vi "MKS VI Probe.vi"() -> ()   [LabVIEW 2015]
doc: "Example VI that demonstrates all library features."
uses:
  PL MKS VI Probe.lvclass
panel:
  in  "baud rate":u32(ring)=19200 items=["300"=300, "600"=600, "1200"=1200, "2400"=2400, "4800"=4800, "9600"=9600, "19200"=19200, "38400"=38400, "76800"=76800, "115200"=115200]
  in  "read software revision":bool
  out "Preact, var":dbl
  out "Pact, W":dbl
  out "Prev, W":dbl
  out "Pfwd, W":dbl
  out "|Z|, Ohm":dbl
  out "Irms, A":dbl
  out "Urms, V":dbl
  out "phase, °":dbl
  in  "save parameters to EEPROM":bool
  out "frequency scan in progress":bool
  in  "Tab Control":enum32{"Frequency scan", "FFT", "Waveforms"}(tab)
  in  "frequency scan parameters":enum32{"range", "array"}(tab)
  in  "frequency range":T1={"start, Hz"=1000000, "stop, Hz"=10000000, "step, Hz"=1000000} {"step, Hz" format="%.0p"; "stop, Hz" format="%.0p"; "start, Hz" format="%.0p"}
  in  "frequency array":u32[](array[numeric]) format="%.0p"
  in  "frequency scan":bool
  out "frequency scan graph":cluster{u32[], dbl[]}[](graph)
  out "frequency scan timeout, ms":u32
  in  "read FFT":bool
  out "FFT graph":T2(graph)
  in  "read waveforms":bool
  out "waveform graph":T3(graph)
  in  "buffers":u16(ring) items=["all on", "oscilloscope on", "spectrum on", "all off"]
  in  "acquisition time, ms":u16(ring) items=["4.08", "6.08", "12.20", "20.96", "42.61", "85.20", "170.40", "348.60", "687.20"]
  in  "averaging":u16(ring) items=["1", "2", "4", "8", "16", "32", "64", "128"]
  in  "end address":u32
  in  "start address":u32
  in  "frequency, Hz":u32=1000000 format="%.0p"
  in  "read firmware checksum":bool
  out "VI Probe":refnum<class "PL MKS VI Probe.lvclass">
  in  "port":refnum<visa-resource-name>
  out "error":errorcluster
  in  "stop":bool
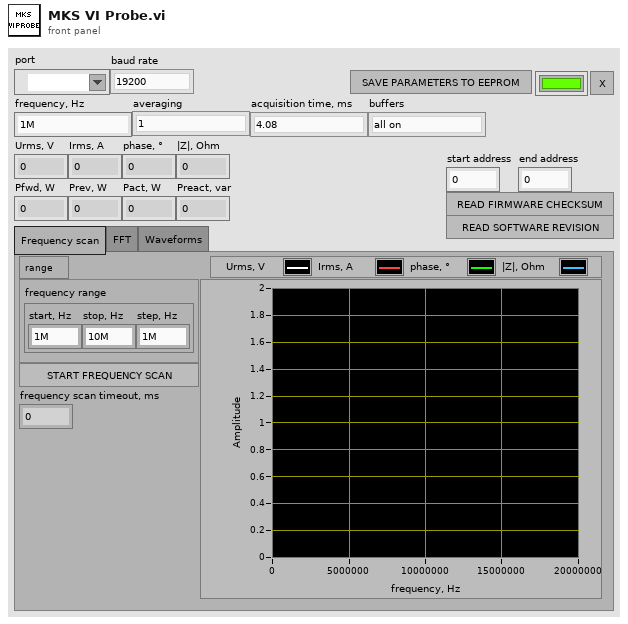
[diagram p1: front panel]
types:
  T1 = cluster{"start, Hz":u32, "stop, Hz":u32, "step, Hz":u32}
  T2 = cluster{"f, Hz":dbl, "df, Hz":dbl, "magnitude, dB":dbl[][]}
  T3 = cluster{"t0, s":dbl, "dt, s":dbl, "U, V":dbl[][]}
  T4 = cluster{"frequency, Hz":u32, "time, s":dbl, "status":cluster{"rf on":bool, "time overflow":bool, "avarage data valid":bool, "below scan threshold":bool, "computational overflow":bool}, "Urms, V":dbl, "Irms, A":dbl, "phase difference, °":dbl, "|Z|, Ohm":dbl}
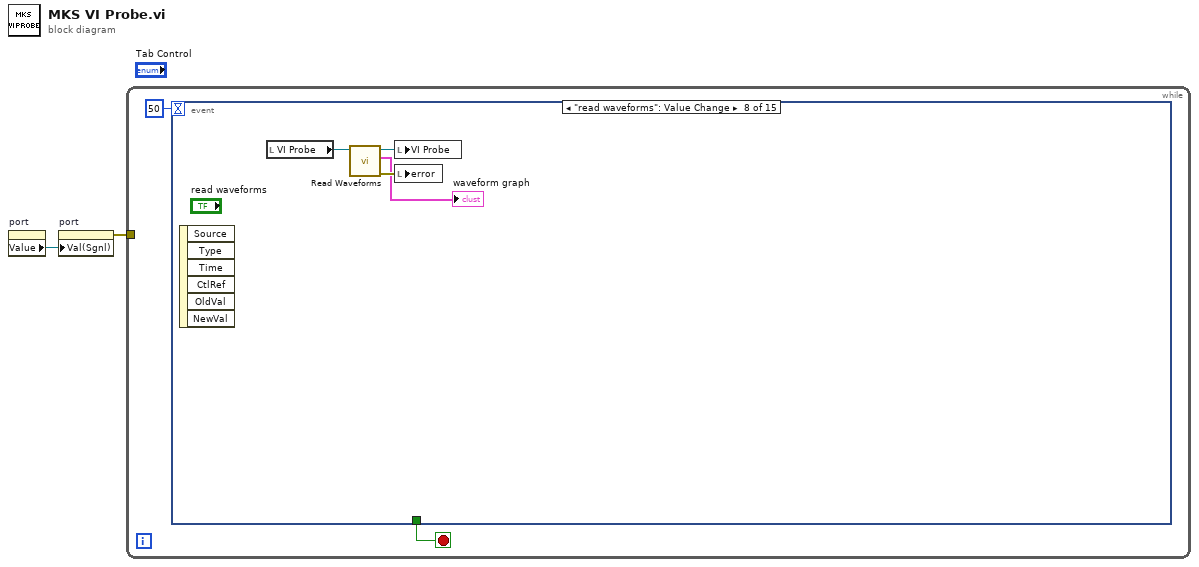
[diagram p0: block diagram]
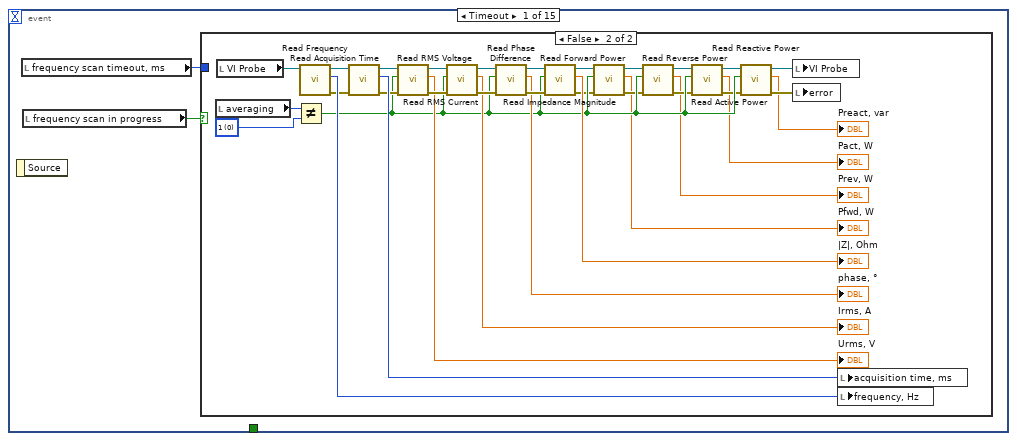
[diagram p2: hidden frame]
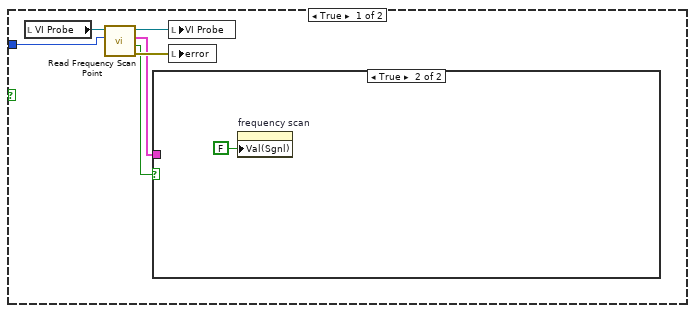
[diagram p3: hidden frame]
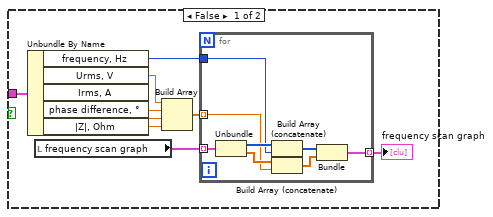
[diagram p4: hidden frame]
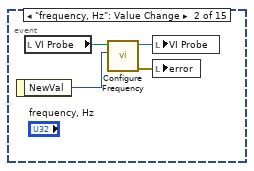
[diagram p5: hidden frame]
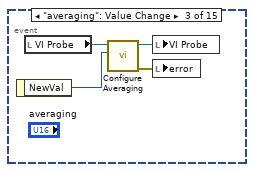
[diagram p6: hidden frame]
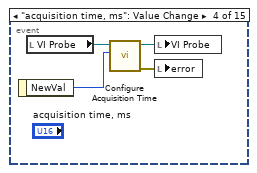
[diagram p7: hidden frame]
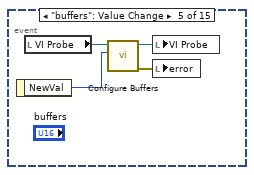
[diagram p8: hidden frame]
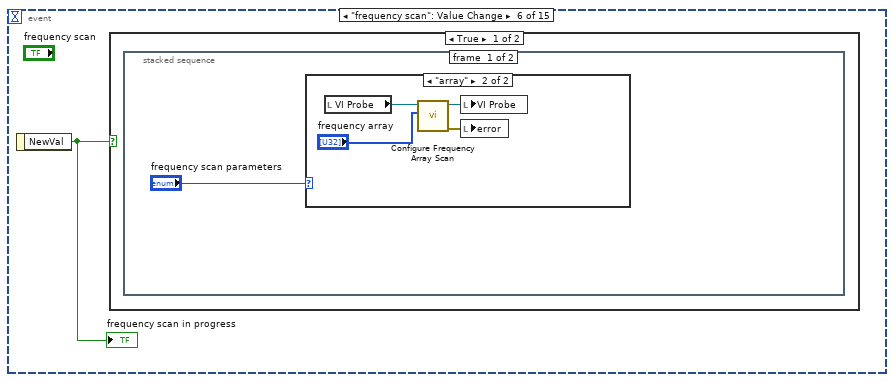
[diagram p9: hidden frame]
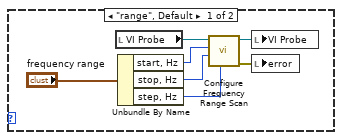
[diagram p10: hidden frame]
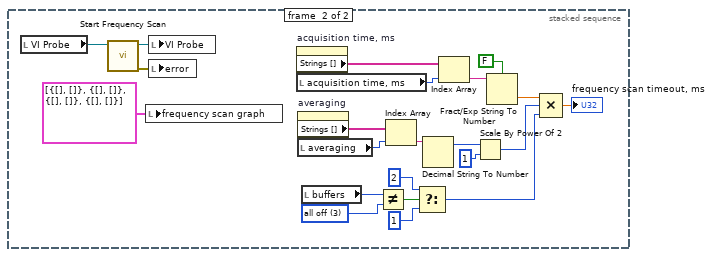
[diagram p11: hidden frame]
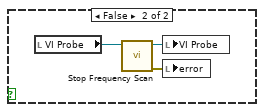
[diagram p12: hidden frame]
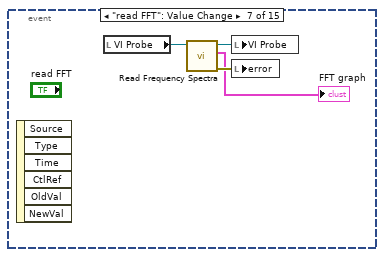
[diagram p13: hidden frame]
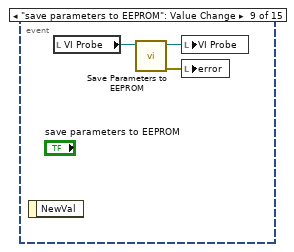
[diagram p14: hidden frame]
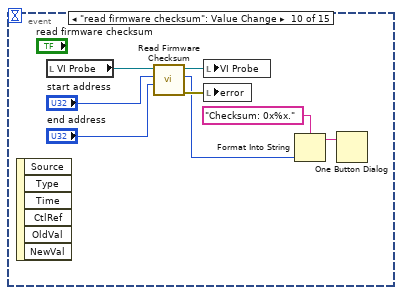
[diagram p15: hidden frame]
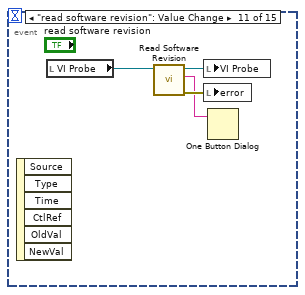
[diagram p16: hidden frame]
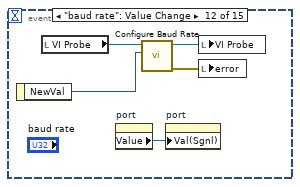
[diagram p17: hidden frame]
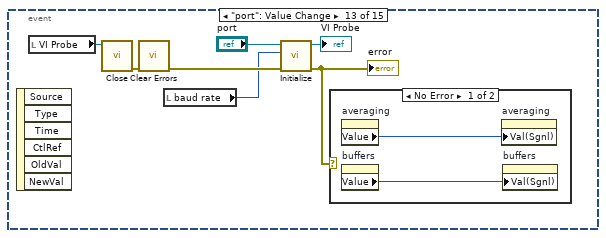
[diagram p18: hidden frame]
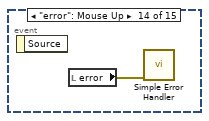
[diagram p20: hidden frame]
diagram:
  n1 = property on="port" class="VISAName"() -> ("Value"=w1:refnum<visa-resource-name>)  [unwired: 2 in, 2 out]
  n2 = property on="port" class="VISAName"("Val(Sgnl)"=w1) -> (error out=w2:errorcluster)  [unwired: 2 in, 1 out]
  n3 = while {
    tunnel: w2 -> [_]
    stop <- w3 stop-if-true
    n4 = event shown="[7] \"read waveforms\": Value Change" {
      selector: _ -> [_ _ _ _ _ _ _ _ _ _ _ _ _ _ _]
      dyn-events: _ -> [_ _ _ _ _ _ _ _ _ _ _ _ _ _ _]
      timeout: 50 -> [_ _ _ _ _ _ _ _ _ _ _ _ _ _ _]
      tunnel: [_ _ _ _ _ _ _ _ _ _ _ _ _ _ TRUE ("stop")] -> w3
      event Timeout {
        n5 = event-data() -> ()  [unwired: 1 in, 1 out]
        n6 = local read "frequency scan timeout, ms"() -> (w5:u32)
        n7 = local read "frequency scan in progress"() -> (w6:bool)
        n8 = case shown="False" w6 {
          tunnel: w5 -> [w9 _]
          frame True {
            n9 = local read "VI Probe"() -> (w12:refnum<class "PL MKS VI Probe.lvclass">)
            n10 = call "Read Frequency Scan Point.vi"("additional timeout, ms (0)"=w9, "VI Probe in"=w12) -> ("error out"=w10:errorcluster, "end of scan"=w7:bool, "scan point"=w8:T4, "VI Probe out"=w11:refnum<class "PL MKS VI Probe.lvclass">)  [unwired: 6 in]
            n11 = case shown="True" w7 {
              tunnel: w8 -> [w21 _]
              frame False {
                n12 = Unbundle By Name(w21) -> ("frequency, Hz"=w14:u32, "Urms, V"=w19:dbl, "Irms, A"=w18:dbl, "phase difference, °"=w17:dbl, "|Z|, Ohm"=w16:dbl)
                n13 = local read "frequency scan graph"() -> (w20:cluster{u32[], dbl[]}[])
                n14 = Build Array(w19, w18, w17, w16) -> (w15:dbl[])
                n15 = for {
                  tunnel: w20 -> [w29] mode=indexing
                  tunnel: w15 -> [w25] mode=indexing
                  tunnel: w14 -> [w26]
                  tunnel: [w22] -> w13 mode=indexing
                  n16 = Unbundle(w29) -> (w28:u32[], w27:dbl[])
                  n17 = Build Array (concatenate)(w28, w26) -> (w24:u32[])
                  n18 = Build Array (concatenate)(w27, w25) -> (w23:dbl[])
                  n19 = Bundle(w24, w23) -> (w22:cluster{u32[], dbl[]})  [unwired: 1 in]
                }
                "frequency scan graph" <- w13
              }
              frame True {
                n20 = property on="frequency scan" class="Bool (strict)"("Val(Sgnl)"=FALSE ("Value (Signaling)")) -> ()  [unwired: 2 in, 2 out]
              }
            }
            n21 = local write "VI Probe"(w11) -> ()
            n22 = local write "error"(w10) -> ()
          }
          frame False {
            w59 = u16 0 items=["1", "2", "4", "8", "16", "32", "64", "128"] ("averaging")
            n23 = local read "averaging"() -> (w58:u16)
            n24 = local read "VI Probe"() -> (w64:refnum<class "PL MKS VI Probe.lvclass">)
            n25 = Not Equal?(x=w58, y=w59) -> (x != y?=w45:bool)
            n26 = call "Read Frequency.vi"("VI Probe in"=w64) -> ("error out"=w61:errorcluster, "frequency, Hz"=w63:u32, "VI Probe out"=w62:refnum<class "PL MKS VI Probe.lvclass">)  [unwired: 8 in]
            n27 = call "Read Acquisition Time.vi"("error in (no error)"=w61, "VI Probe in"=w62) -> ("error out"=w50:errorcluster, "acquisition time, ms"=w60:u16, "VI Probe out"=w57:refnum<class "PL MKS VI Probe.lvclass">)  [unwired: 7 in]
            n28 = call "Read RMS Voltage.vi"("error in (no error)"=w50, "average (false)"=w45, "VI Probe in"=w57) -> ("error out"=w51:errorcluster, "Urms, V"=→"Urms, V":dbl, "VI Probe out"=w56:refnum<class "PL MKS VI Probe.lvclass">)  [unwired: 6 in]
            n29 = call "Read RMS Current.vi"("error in (no error)"=w51, "average (false)"=w45, "VI Probe in"=w56) -> ("error out"=w52:errorcluster, "Irms, A"=→"Irms, A":dbl, "VI Probe out"=w55:refnum<class "PL MKS VI Probe.lvclass">)  [unwired: 6 in]
            n30 = call "Read Phase Difference.vi"("error in (no error)"=w52, "average (false)"=w45, "VI Probe in"=w55) -> ("error out"=w53:errorcluster, "phase difference, °"=→"phase, °":dbl, "VI Probe out"=w54:refnum<class "PL MKS VI Probe.lvclass">)  [unwired: 6 in]
            n31 = call "Read Impedance Magnitude.vi"("error in (no error)"=w53, "average (false)"=w45, "VI Probe in"=w54) -> ("error out"=w35:errorcluster, "|Z|, Ohm"=→"|Z|, Ohm":dbl, "VI Probe out"=w44:refnum<class "PL MKS VI Probe.lvclass">)  [unwired: 6 in]
            n32 = call "Read Forward Power.vi"("error in (no error)"=w35, "average (false)"=w45, "VI Probe in"=w44) -> ("error out"=w36:errorcluster, "Pfwd, W"=→"Pfwd, W":dbl, "VI Probe out"=w43:refnum<class "PL MKS VI Probe.lvclass">)  [unwired: 6 in]
            n33 = call "Read Reverse Power.vi"("error in (no error)"=w36, "average (false)"=w45, "VI Probe in"=w43) -> ("error out"=w37:errorcluster, "Prev, W"=→"Prev, W":dbl, "VI Probe out"=w42:refnum<class "PL MKS VI Probe.lvclass">)  [unwired: 6 in]
            n34 = call "Read Active Power.vi"("error in (no error)"=w37, "average (false)"=w45, "VI Probe in"=w42) -> ("error out"=w38:errorcluster, "Pact, W"=→"Pact, W":dbl, "VI Probe out"=w41:refnum<class "PL MKS VI Probe.lvclass">)  [unwired: 6 in]
            n35 = call "Read Reactive Power.vi"("error in (no error)"=w38, "average (false)"=w45, "VI Probe in"=w41) -> ("error out"=w39:errorcluster, "Preact, var"=→"Preact, var":dbl, "VI Probe out"=w40:refnum<class "PL MKS VI Probe.lvclass">)  [unwired: 6 in]
            n36 = local write "VI Probe"(w40) -> ()
            n37 = local write "error"(w39) -> ()
            n38 = local write "acquisition time, ms"(w60) -> ()
            n39 = local write "frequency, Hz"(w63) -> ()
          }
        }
      }
      event "frequency, Hz": Value Change {
        n40 = event-data() -> ("NewVal"=w65:u32)  [unwired: 1 in]
        n41 = local read "VI Probe"() -> (w68:refnum<class "PL MKS VI Probe.lvclass">)
        n42 = call "Configure Frequency.vi"("frequency, Hz"=w65, "VI Probe in"=w68) -> ("error out"=w66:errorcluster, "VI Probe out"=w67:refnum<class "PL MKS VI Probe.lvclass">)  [unwired: 8 in]
        n43 = local write "VI Probe"(w67) -> ()
        n44 = local write "error"(w66) -> ()
      }
      event "averaging": Value Change {
        n45 = event-data() -> ("NewVal"=w69:u16)  [unwired: 1 in]
        n46 = local read "VI Probe"() -> (w72:refnum<class "PL MKS VI Probe.lvclass">)
        n47 = call "Configure Averaging.vi"("number of points"=w69, "VI Probe in"=w72) -> ("error out"=w70:errorcluster, "VI Probe out"=w71:refnum<class "PL MKS VI Probe.lvclass">)  [unwired: 8 in]
        n48 = local write "VI Probe"(w71) -> ()
        n49 = local write "error"(w70) -> ()
      }
      event "acquisition time, ms": Value Change {
        n50 = event-data() -> ("NewVal"=w73:u16)  [unwired: 1 in]
        n51 = local read "VI Probe"() -> (w76:refnum<class "PL MKS VI Probe.lvclass">)
        n52 = call "Configure Acquisition Time.vi"("acquisition time, ms"=w73, "VI Probe in"=w76) -> ("error out"=w74:errorcluster, "VI Probe out"=w75:refnum<class "PL MKS VI Probe.lvclass">)  [unwired: 8 in]
        n53 = local write "VI Probe"(w75) -> ()
        n54 = local write "error"(w74) -> ()
      }
      event "buffers": Value Change {
        n55 = event-data() -> ("NewVal"=w77:u16)  [unwired: 1 in]
        n56 = local read "VI Probe"() -> (w80:refnum<class "PL MKS VI Probe.lvclass">)
        n57 = call "Configure Buffers.vi"("mode"=w77, "VI Probe in"=w80) -> ("error out"=w78:errorcluster, "VI Probe out"=w79:refnum<class "PL MKS VI Probe.lvclass">)  [unwired: 8 in]
        n58 = local write "VI Probe"(w79) -> ()
        n59 = local write "error"(w78) -> ()
      }
      event "frequency scan": Value Change {
        n60 = event-data() -> ("NewVal"=w81:bool)  [unwired: 1 in]
        "frequency scan in progress" <- w81
        n61 = case shown="True" w81 {
          frame True {
            n62 = stacked-sequence {
              frame #0 {
                n63 = case shown="\"array\"" "frequency scan parameters" {
                  frame "range", Default {
                    n64 = local read "VI Probe"() -> (w88:refnum<class "PL MKS VI Probe.lvclass">)
                    n65 = Unbundle By Name("frequency range") -> ("start, Hz"=w87:u32, "stop, Hz"=w86:u32, "step, Hz"=w85:u32)
                    n66 = call "Configure Frequency Range Scan.vi"("step, Hz"=w85, "stop, Hz"=w86, "start, Hz"=w87, "VI Probe in"=w88) -> ("error out"=w84:errorcluster, "VI Probe out"=w83:refnum<class "PL MKS VI Probe.lvclass">)  [unwired: 6 in]
                    n67 = local write "VI Probe"(w83) -> ()
                    n68 = local write "error"(w84) -> ()
                  }
                  frame "array" {
                    n69 = local read "VI Probe"() -> (w93:refnum<class "PL MKS VI Probe.lvclass">)
                    n70 = call "Configure Frequency Array Scan.vi"("frequencies, Hz"="frequency array", "VI Probe in"=w93) -> ("error out"=w92:errorcluster, "VI Probe out"=w91:refnum<class "PL MKS VI Probe.lvclass">)  [unwired: 8 in]
                    n71 = local write "VI Probe"(w91) -> ()
                    n72 = local write "error"(w92) -> ()
                  }
                }
              }
              frame #1 {
                w95 = u16 3 items=["all on", "oscilloscope on", "spectrum on", "all off"] ("buffers")
                n73 = local read "VI Probe"() -> (w114:refnum<class "PL MKS VI Probe.lvclass">)
                n74 = call "Start Frequency Scan.vi"("VI Probe in"=w114) -> ("error out"=w112:errorcluster, "VI Probe out"=w113:refnum<class "PL MKS VI Probe.lvclass">)  [unwired: 9 in]
                n75 = local write "frequency scan graph"(cluster{u32[], dbl[]}[] [{[], []}, {[], []}, {[], []}, {[], []}] ("frequency scan graph")) -> ()
                n76 = local write "VI Probe"(w113) -> ()
                n77 = local write "error"(w112) -> ()
                n78 = property on="acquisition time, ms" class="Ring (strict)"() -> ("Strings []"=w104:string[])  [unwired: 2 in, 2 out]
                n79 = local read "acquisition time, ms"() -> (w105:u16)
                n80 = property on="averaging" class="Ring (strict)"() -> ("Strings []"=w99:string[])  [unwired: 2 in, 2 out]
                n81 = local read "averaging"() -> (w100:u16)
                n82 = local read "buffers"() -> (w94:u16)
                n83 = Not Equal?(x=w94, y=w95) -> (x != y?=w96:bool)
                n84 = Index Array(array=w99, index=w100) -> (element=w101:string)
                n85 = Select(t=u32 2 ("additional timeout, ms (0)"), s=w96, f=u32 1 ("additional timeout, ms (0)")) -> (s? t:f=w110:u32)
                n86 = Decimal String To Number(string=w101) -> (offset past number=w102:i32)  [unwired: 2 in, 1 out]
                n87 = Index Array(array=w104, index=w105) -> (element=w106:string)
                n88 = Scale By Power Of 2(n=w102, x=u32 1) -> (x*2^n=w109:u32)
                n89 = Fract/Exp String To Number(use system decimal point (T)=FALSE, string=w106) -> (number=w108:dbl)  [unwired: 2 in, 1 out]
                n90 = Compound Arithmetic op=MULTIPLY(w108, w109, w110) -> (→"frequency scan timeout, ms":dbl)
              }
            }
          }
          frame False {
            n91 = local read "VI Probe"() -> (w118:refnum<class "PL MKS VI Probe.lvclass">)
            n92 = call "Stop Frequency Scan.vi"("VI Probe in"=w118) -> ("error out"=w116:errorcluster, "VI Probe out"=w117:refnum<class "PL MKS VI Probe.lvclass">)  [unwired: 9 in]
            n93 = local write "VI Probe"(w117) -> ()
            n94 = local write "error"(w116) -> ()
          }
        }
      }
      event "read FFT": Value Change {
        n95 = event-data() -> ()  [unwired: 1 in, 6 out]
        n96 = local read "VI Probe"() -> (w122:refnum<class "PL MKS VI Probe.lvclass">)
        n97 = call "Read Frequency Spectra.vi"("VI Probe in"=w122) -> ("error out"=w120:errorcluster, "spectra"=→"FFT graph":T2, "VI Probe out"=w121:refnum<class "PL MKS VI Probe.lvclass">)  [unwired: 8 in]
        n98 = local write "VI Probe"(w121) -> ()
        n99 = local write "error"(w120) -> ()
      }
      event "read waveforms": Value Change {
        n100 = event-data() -> ()  [unwired: 1 in, 6 out]
        n101 = local read "VI Probe"() -> (w126:refnum<class "PL MKS VI Probe.lvclass">)
        n102 = call "Read Waveforms.vi"("VI Probe in"=w126) -> ("error out"=w124:errorcluster, "waveforms"=→"waveform graph":T3, "VI Probe out"=w125:refnum<class "PL MKS VI Probe.lvclass">)  [unwired: 8 in]
        n103 = local write "VI Probe"(w125) -> ()
        n104 = local write "error"(w124) -> ()
      }
      event "save parameters to EEPROM": Value Change {
        n105 = event-data() -> ()  [unwired: 1 in, 1 out]
        n106 = local read "VI Probe"() -> (w129:refnum<class "PL MKS VI Probe.lvclass">)
        n107 = call "Save Parameters to EEPROM.vi"("VI Probe in"=w129) -> ("error out"=w127:errorcluster, "VI Probe out"=w128:refnum<class "PL MKS VI Probe.lvclass">)  [unwired: 9 in]
        n108 = local write "VI Probe"(w128) -> ()
        n109 = local write "error"(w127) -> ()
      }
      event "read firmware checksum": Value Change {
        n110 = event-data() -> ()  [unwired: 1 in, 6 out]
        n111 = local read "VI Probe"() -> (w135:refnum<class "PL MKS VI Probe.lvclass">)
        n112 = call "Read Firmware Checksum.vi"("end address (all)"="end address", "start address (0)"="start address", "VI Probe in"=w135) -> ("error out"=w137:errorcluster, "checksum"=w132:u32, "VI Probe out"=w136:refnum<class "PL MKS VI Probe.lvclass">)  [unwired: 6 in]
        n113 = local write "VI Probe"(w136) -> ()
        n114 = local write "error"(w137) -> ()
        n115 = Format Into String(format string="Checksum: 0x%x.", w132) -> (resulting string=w134:string)  [unwired: 2 in, 1 out]
        n116 = One Button Dialog(message=w134) -> ()  [unwired: 1 in, 1 out]
      }
      event "read software revision": Value Change {
        n117 = event-data() -> ()  [unwired: 1 in, 6 out]
        n118 = local read "VI Probe"() -> (w139:refnum<class "PL MKS VI Probe.lvclass">)
        n119 = call "Read Software Revision.vi"("VI Probe in"=w139) -> ("error out"=w141:errorcluster, "software revision"=w138:string, "VI Probe out"=w140:refnum<class "PL MKS VI Probe.lvclass">)  [unwired: 8 in]
        n120 = local write "VI Probe"(w140) -> ()
        n121 = local write "error"(w141) -> ()
        n122 = One Button Dialog(message=w138) -> ()  [unwired: 1 in, 1 out]
      }
      event "baud rate": Value Change {
        n123 = event-data() -> ("NewVal"=w143:u32)  [unwired: 1 in]
        n124 = local read "VI Probe"() -> (w146:refnum<class "PL MKS VI Probe.lvclass">)
        n125 = property on="port" class="VISAName"() -> ("Value"=w142:refnum<visa-resource-name>)  [unwired: 2 in, 2 out]
        n126 = call "Configure Baud Rate.vi"("baud rate"=w143, "VI Probe in"=w146) -> ("error out"=w144:errorcluster, "VI Probe out"=w145:refnum<class "PL MKS VI Probe.lvclass">)  [unwired: 8 in]
        n127 = property on="port" class="VISAName"("Val(Sgnl)"=w142) -> ()  [unwired: 2 in, 2 out]
        n128 = local write "VI Probe"(w145) -> ()
        n129 = local write "error"(w144) -> ()
      }
      event "port": Value Change {
        n130 = event-data() -> ()  [unwired: 1 in, 6 out]
        n131 = local read "VI Probe"() -> (w153:refnum<class "PL MKS VI Probe.lvclass">)
        n132 = call "Close.vi"("VI Probe in"=w153) -> ("error out"=w151:errorcluster)  [unwired: 10 in]
        n133 = call <vilib>:"Clear Errors.vi"("error in (no error)"=w151) -> ("error out"=w152:errorcluster)  [unwired: 5 in, 1 out]
        n134 = local read "baud rate"() -> (w148:u32)
        n135 = call "Initialize.vi"("error in (no error)"=w152, "baud rate (19200)"=w148, "port"="port") -> ("error out"=w147:errorcluster, "VI Probe out"=→"VI Probe":refnum<class "PL MKS VI Probe.lvclass">)  [unwired: 7 in]
        "error" <- w147
        n136 = case shown="No Error" w147 {
          frame No Error {
            n137 = property on="averaging" class="Ring (strict)"() -> ("Value"=w155:u16)  [unwired: 2 in, 2 out]
            n138 = property on="buffers" class="Ring (strict)"() -> ("Value"=w154:u16)  [unwired: 2 in, 2 out]
            n139 = property on="averaging" class="Ring (strict)"("Val(Sgnl)"=w155) -> ()  [unwired: 2 in, 2 out]
            n140 = property on="buffers" class="Ring (strict)"("Val(Sgnl)"=w154) -> ()  [unwired: 2 in, 2 out]
          }
          frame Error {
          }
        }
      }
      event "error": Mouse Up {
        n141 = event-data() -> ()  [unwired: 1 in, 1 out]
        n142 = local read "error"() -> (w156:errorcluster)
        n143 = call <vilib>:"Simple Error Handler.vi"("error in (no error)"=w156) -> ()  [unwired: 4 in, 5 out]
      }
      event "stop": Value Change {
        n144 = event-data() -> ()  [unwired: 1 in, 1 out]
        n145 = local read "VI Probe"() -> (w158:refnum<class "PL MKS VI Probe.lvclass">)
        n146 = call "Close.vi"("VI Probe in"=w158) -> ("error out"=w157:errorcluster)  [unwired: 10 in]
        n147 = call <vilib>:"Clear Errors.vi"("error in (no error)"=w157) -> ()  [unwired: 5 in, 2 out]
      }
    }
  }
